vi "LVClass_HasoSlopes Get Parameters.vi"(0 "HasoSlopes in":refnum<class "HasoSlopes.lvclass">, 11 "error in (no error)":errorcluster) -> (4 "HasoSlopes out":refnum<class "HasoSlopes.lvclass">, 8 "Pamameter":T1, 15 "error out":errorcluster)   [LabVIEW 2020, in "HasoSlopes.lvclass"]
doc: "Compute HasoSlopes geometric parameters.\n\n--------------------------------------------------------------------------------\n\n<B>HasoSlopesIn </B> : HasoSlopes object.\n<B>HasoSlopesOut </B> : HasoSlopes object.\n<B>tiltX_mrad </B> : x tilt (mrad).\n<B>tiltY_mrad </B> : y tilt (mrad).\n<B>radius_mm </B> : radius (mm).\n<B>focus_Xpos_mm </B> : x focus position (mm).\n<B>focus_Ypos_mm </B> : y focus position (mm).\n<B>astig_angle_rad </B> : astgimatism angle (rad).\n<B>sagittal_focal_length_mm </B> : sagittal focal length (mm).\n<B>tangential_focal_length_mm </B> : tangential focal length (mm).\n<B>ErrorIn </B> : Error\n<B>ErrorOut </B> : Error\n\n--------------------------------------------------------------------------------"
uses:
  HasoSlopes.lvclass
  HasoSlopes.lvclass/HasoSlopes.ctl
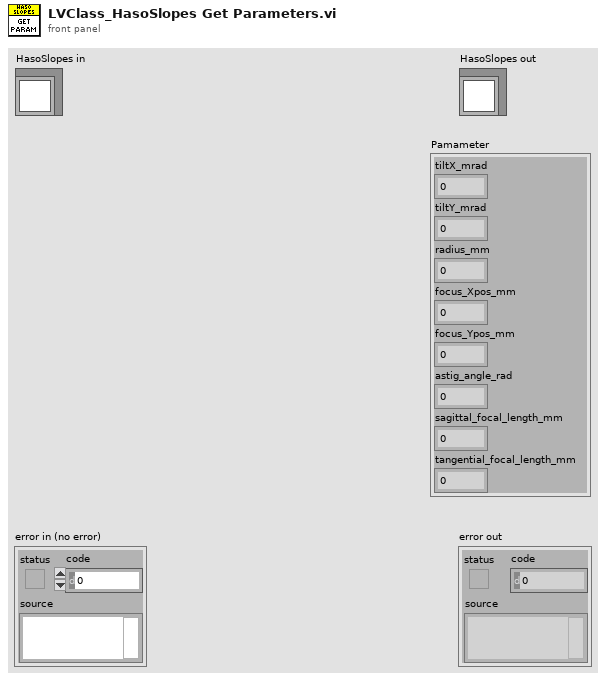
[diagram p1: front panel]
types:
  T1 = cluster{"tiltX_mrad":sgl, "tiltY_mrad":dbl, "radius_mm":sgl, "focus_Xpos_mm":sgl, "focus_Ypos_mm":sgl, "astig_angle_rad":sgl, "sagittal_focal_length_mm":sgl, "tangential_focal_length_mm":sgl}
  T2 = typedef "ClassID.ctl" = i64
  T3 = cluster{"tiltX_mrad":sgl, "tiltY_mrad":sgl, "radius_mm":sgl, "focus_Xpos_mm":sgl, "focus_Ypos_mm":sgl, "astig_angle_rad":sgl, "sagittal_focal_length_mm":sgl, "tangential_focal_length_mm":sgl}
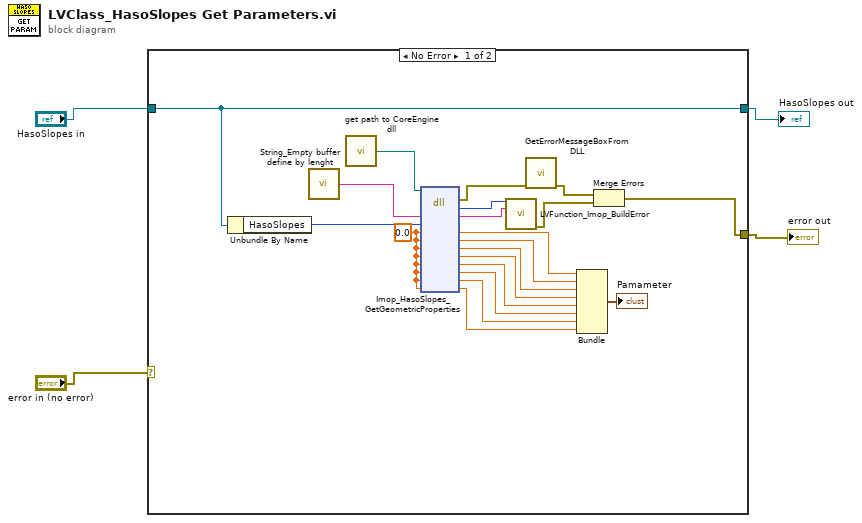
[diagram p0: block diagram]
diagram:
  n1 = case shown="No Error" "error in (no error)" {
    selector: "error in (no error)" -> [_ w26]
    tunnel: [w5 w26] -> w1
    tunnel: [w10 w25] -> w2
    tunnel: "HasoSlopes in" -> [w10 w25]
    frame No Error {
      w19 = sgl 0.0 ("tiltX_mrad")
      n2 = Unbundle By Name(w10) -> ("HasoSlopes"=w9:T2)
      n3 = call "String_Empty buffer define by lenght.vi"() -> ("Empty buffer"=w22:string)  [unwired: 1 in]
      n4 = call "get path to CoreEngine dll.vi"() -> ("path to wavekit library"=w21:path)  [unwired: 14 in, 1 out]
      n5 = dll-call lib="D:/FLE/0.Code/CoreEngine4_Suite/LV2011_interface/DLLs/c_interface_vc100.dll" fn="Imop_HasoSlopes_GetGeometricProperties"(path in=w21, "message"=w22, "objet"=w9, "tiltX_mrad"=w19, "tiltY_mrad"=w19, "radius_mm"=w19, "focus_Xpos_mm"=w19, "focus_Ypos_mm"=w19, "astig_angle_rad"=w19, "sagittal_focal_length_mm"=w19, "tangential_focal_length_mm"=w19) -> (error out=w20:errorcluster, "return type"=w24:i32, "message"=w23:string, "tiltX_mrad"=w18:sgl, "tiltY_mrad"=w8:sgl, "radius_mm"=w17:sgl, "focus_Xpos_mm"=w16:sgl, "focus_Ypos_mm"=w15:sgl, "astig_angle_rad"=w14:sgl, "sagittal_focal_length_mm"=w13:sgl, "tangential_focal_length_mm"=w12:sgl)  [unwired: 3 in, 1 out]
      n6 = call "LVFunction_Imop_BuildError.vi"("code"=w24, "String to Prepend to source (\"\")"=w23) -> ("error out"=w6:errorcluster)  [unwired: 13 in]
      n7 = call "GetErrorMessageBoxFromDLL.vi"("error IN"=w20) -> ("error OUT"=w7:errorcluster)  [unwired: 10 in]
      n8 = Bundle("tiltX_mrad"=w18, "tiltY_mrad"=w8, "radius_mm"=w17, "focus_Xpos_mm"=w16, "focus_Ypos_mm"=w15, "astig_angle_rad"=w14, "sagittal_focal_length_mm"=w13, "tangential_focal_length_mm"=w12) -> (→"Pamameter":T3)  [unwired: 1 in]
      n9 = Merge Errors(w7, w6) -> (w5:errorcluster)
    }
    frame Error {
    }
  }
  "error out" <- w1
  "HasoSlopes out" <- w2
